vi "SplitByChannelType.vi"(8 "error in (no error)":errorcluster, 11 "ScriptEventList in":refnum<class "ScriptEventList.lvclass">) -> (0 "error out":errorcluster, 2 "ScriptLists":T1, 3 "ScriptEventList out":refnum<class "ScriptEventList.lvclass">)   [LabVIEW 2011, in "Tools.lvlib" / "Scripting.lvlib" / "ScriptEventList.lvclass"]
uses:
  ScriptEventList.lvclass
  ScriptEvent.lvclass
  ScriptEventList.lvclass/ScriptEventList.ctl
  DatabaseHelpers/Database Objects/Channel/Channel.lvclass
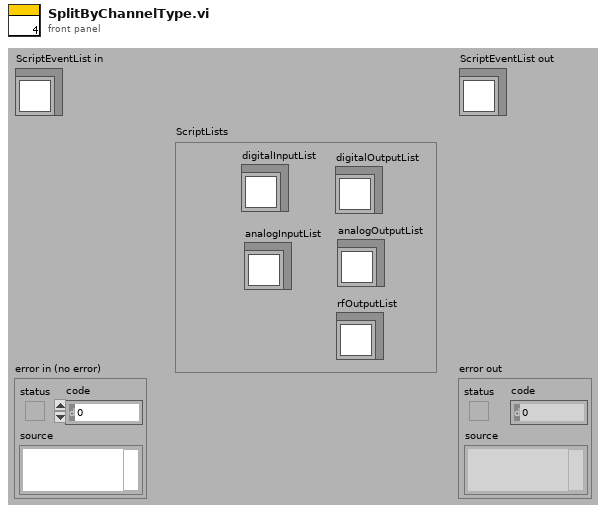
[diagram p1: front panel]
types:
  T1 = cluster{"digitalOutputList":refnum<class "ScriptEventList.lvclass">, "analogOutputList":refnum<class "ScriptEventList.lvclass">, "analogInputList":refnum<class "ScriptEventList.lvclass">, "digitalInputList":refnum<class "ScriptEventList.lvclass">, "rfOutputList":refnum<class "ScriptEventList.lvclass">}
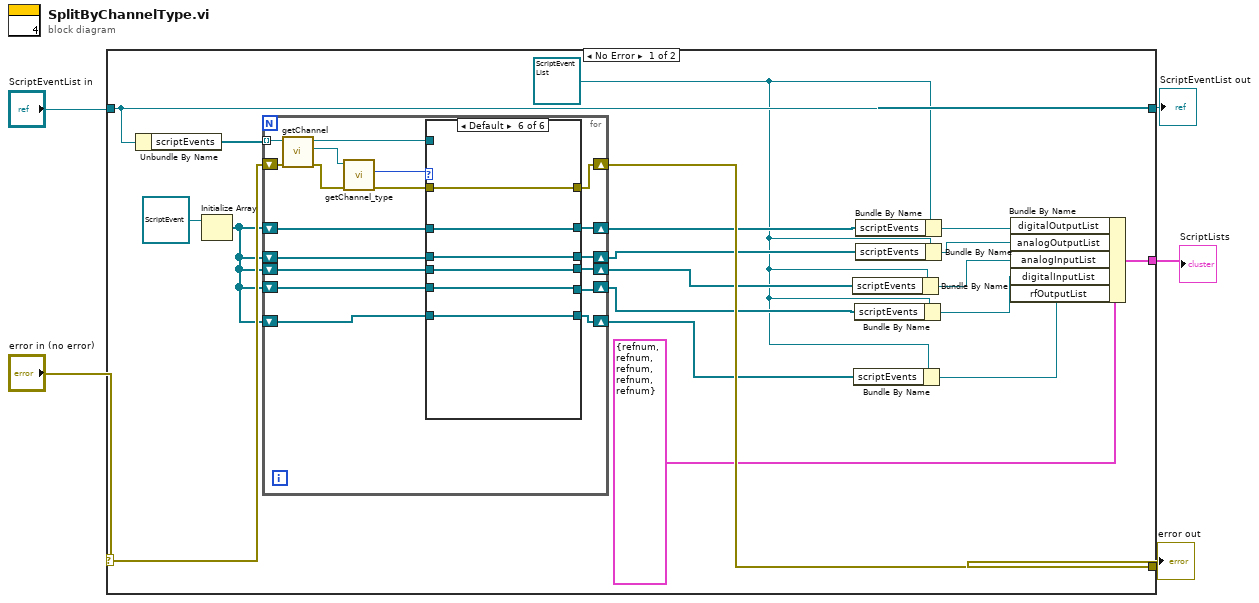
[diagram p0: block diagram]
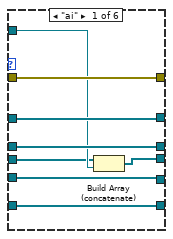
[diagram p2: hidden frame]
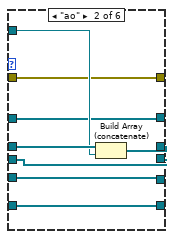
[diagram p3: hidden frame]
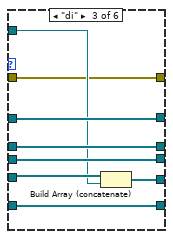
[diagram p4: hidden frame]
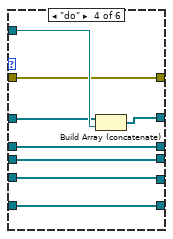
[diagram p5: hidden frame]
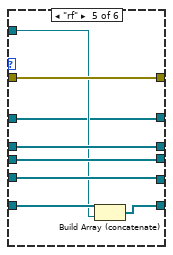
[diagram p6: hidden frame]
diagram:
  n1 = case shown="No Error" "error in (no error)" {
    selector: "error in (no error)" -> [w20 w90]
    tunnel: [w21 w90] -> w4
    tunnel: [w23 w89] -> w2
    tunnel: "ScriptEventList in" -> [w23 w89]
    tunnel: [w6 _] -> w1
    frame No Error {
      w14 = refnum<class "ScriptEventList.lvclass"> refnum ("Tools.lvlib:Scripting.lvlib:ScriptEventList.lvclass")
      n2 = Unbundle By Name(w23) -> ("scriptEvents"=w24:refnum<class "ScriptEvent.lvclass">[])
      n3 = Initialize Array(refnum<class "ScriptEvent.lvclass"> refnum ("Tools.lvlib:Scripting.lvlib:ScriptEvent.lvclass")) -> (w15:refnum<class "ScriptEvent.lvclass">[])  [unwired: 1 in]
      n4 = for {
        tunnel: w24 -> [w42] mode=indexing
        shift-right: [w33] -> w21
        shift-left: w20 -> [w36]
        shift-right: [w35] -> w19
        shift-left: w15 -> [w34]
        shift-right: [w31] -> w18
        shift-left: w15 -> [w32]
        shift-right: [w29] -> w17
        shift-left: w15 -> [w30]
        shift-right: [w27] -> w16
        shift-left: w15 -> [w28]
        shift-right: [w25] -> w13
        shift-left: w15 -> [w26]
        n5 = call-dynamic "getChannel.vi"("error in (no error)"=w36, "ScriptEvent.lvclass in"=w42) -> ("error out"=w40:errorcluster, "Channel.lvclass"=w41:refnum<class "Channel.lvclass">, "ScriptEvent.lvclass out"=w38:refnum<class "ScriptEvent.lvclass">)  [unwired: 7 in]
        n6 = call "getChannel_type.vi"("error in (no error)"=w40, "Channel.lvclass in"=w41) -> ("error out"=w37:errorcluster, "channel_type"=w39:enum16{"ao", "do", "ai", "di", "rf"})  [unwired: 7 in, 1 out]
        n7 = case shown="Default" w39 {
          tunnel: w38 -> [w47 w57 w62 w74 w76 _]
          tunnel: w37 -> [w48 w54 w60 w71 w82 w88]
          tunnel: [w50 w55 w66 w73 w75 w84] -> w35
          tunnel: w34 -> [w50 w55 w66 w72 w75 w84]
          tunnel: [w48 w54 w60 w71 w82 w88] -> w33
          tunnel: w32 -> [w49 w58 w65 w70 w81 w87]
          tunnel: [w49 w56 w65 w70 w81 w87] -> w31
          tunnel: w30 -> [w46 w53 w64 w69 w80 w86]
          tunnel: [w45 w53 w64 w69 w80 w86] -> w29
          tunnel: w28 -> [w44 w52 w63 w68 w79 w85]
          tunnel: [w44 w52 w61 w68 w79 w85] -> w27
          tunnel: w26 -> [w43 w51 w59 w67 w78 w83]
          tunnel: [w43 w51 w59 w67 w77 w83] -> w25
          frame "ai" {
            n8 = Build Array (concatenate)(w46, w47) -> (w45:refnum<class "ScriptEvent.lvclass">[])
          }
          frame "ao" {
            n9 = Build Array (concatenate)(w58, w57) -> (w56:refnum<class "ScriptEvent.lvclass">[])
          }
          frame "di" {
            n10 = Build Array (concatenate)(w63, w62) -> (w61:refnum<class "ScriptEvent.lvclass">[])
          }
          frame "do" {
            n11 = Build Array (concatenate)(w72, w74) -> (w73:refnum<class "ScriptEvent.lvclass">[])
          }
          frame "rf" {
            n12 = Build Array (concatenate)(w78, w76) -> (w77:refnum<class "ScriptEvent.lvclass">[])
          }
          frame Default {
          }
        }
      }
      n13 = Bundle By Name(cluster=w14, "scriptEvents"=w17) -> (w12:refnum<class "ScriptEventList.lvclass">)
      n14 = Bundle By Name(cluster=w14, "scriptEvents"=w13) -> (w11:refnum<class "ScriptEventList.lvclass">)
      n15 = Bundle By Name(cluster=w14, "scriptEvents"=w16) -> (w7:refnum<class "ScriptEventList.lvclass">)
      n16 = Bundle By Name(cluster=w14, "scriptEvents"=w19) -> (w8:refnum<class "ScriptEventList.lvclass">)
      n17 = Bundle By Name(cluster=w14, "scriptEvents"=w18) -> (w9:refnum<class "ScriptEventList.lvclass">)
      n18 = Bundle By Name(cluster=T1 {"digitalOutputList"=refnum, "analogOutputList"=refnum, "analogInputList"=refnum, "digitalInputList"=refnum, "rfOutputList"=refnum} ("ScriptLists"), "digitalOutputList"=w8, "analogOutputList"=w9, "analogInputList"=w12, "digitalInputList"=w7, "rfOutputList"=w11) -> (w6:T1)
    }
    frame Error {
    }
  }
  "error out" <- w4
  "ScriptEventList out" <- w2
  "ScriptLists" <- w1
